vi "Test Process Executor Run.vi"() -> (0 "error out":errorcluster)   [LabVIEW 2025]
doc: "This smoke test verifies that the ProcessExecutor.Run method can successfully start an external process and return without error. The test executes a simple, short-lived system command and asserts only that no error is reported, confirming that process creation, argument serialization, and basic timeout handling are functioning correctly."
uses:
  src/Process Executor/Process Executor.lvclass
  src/Type Definitions/Execution Plan--cluster.ctl
  <vilib>/addons/_JKI Toolkits/Caraya/classes/Test/Test.lvclass
  <vilib>/addons/_JKI Toolkits/Caraya/classes/Assert/Assert.lvclass
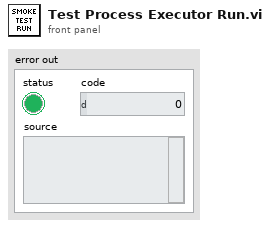
[diagram p1: front panel]
types:
  T1 = typedef "Execution Plan--cluster.ctl" = cluster{"Exe Path":path, "Args":string[], "Timeout":i32}
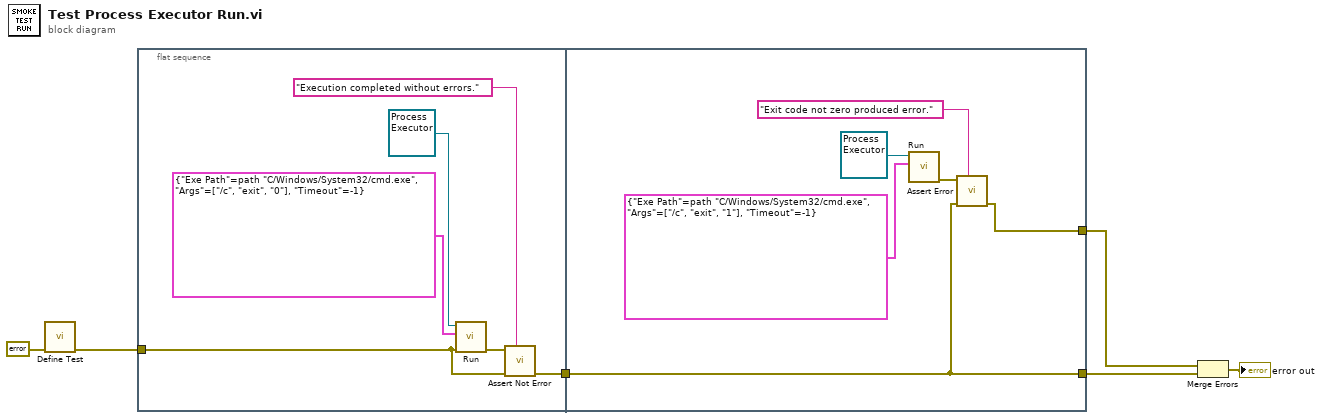
[diagram p0: block diagram]
diagram:
  n1 = call <vilib>:"Define Test.vi"("error in (no error)"=errorcluster {"status"=FALSE, "code"=0, "source"=""}) -> ("error out"=w4:errorcluster)  [unwired: 9 in, 1 out]
  n2 = flat-sequence {
    tunnel: w4 -> [w7]
    tunnel: [w8] -> w2
    tunnel: [w13] -> w3
    tunnel: w2 -> [w13]
    tunnel: [w14] -> w1
    frame #0 {
      n3 = call-dynamic "Run.vi"("error in"=w7, "Execution Plan"=T1 {"Exe Path"=path "C:/Windows/System32/cmd.exe", "Args"=["/c", "exit", "0"], "Timeout"=-1}, "Process Executor in"=refnum<class "Process Executor.lvclass"> refnum) -> ("error out"=w12:errorcluster)  [unwired: 7 in, 1 out]
      n4 = call <vilib>:"Assert Not Error.vi"("Label"="Execution completed without errors.", "error in (no error)"=w7, "Not Error?"=w12) -> ("error out"=w8:errorcluster)  [unwired: 7 in, 1 out]
    }
    frame #1 {
      n5 = call-dynamic "Run.vi"("Execution Plan"=T1 {"Exe Path"=path "C:/Windows/System32/cmd.exe", "Args"=["/c", "exit", "1"], "Timeout"=-1}, "Process Executor in"=refnum<class "Process Executor.lvclass"> refnum) -> ("error out"=w18:errorcluster)  [unwired: 8 in, 1 out]
      n6 = call <vilib>:"Assert Error.vi"("Label"="Exit code not zero produced error.", "error in (no error)"=w13, "Error?"=w18) -> ("error out"=w14:errorcluster)  [unwired: 7 in, 1 out]
    }
  }
  n7 = Merge Errors(w1, w3) -> (→"error out":errorcluster)
